vi "ADIS16448_CRC.vi"() -> (2 "CRC16-ADIS":u16, 10 "16-bit Array":i16[](array[numeric])=[15, -8, 10, -447, -52, 1110, 551, -605, -3054, -16068, -148])   [LabVIEW 2017]
panel:
  out "8-bit Array":u8[](array[numeric])
  # "This vi calculates a CRC16 check on data generated from an \nADIS16448 IMU when using burst mode (MSC_CTRL[4] = 1). \nThis implementation is a variant of the CCITT X.25 spec.\n\nJuan Chong - December 2017"
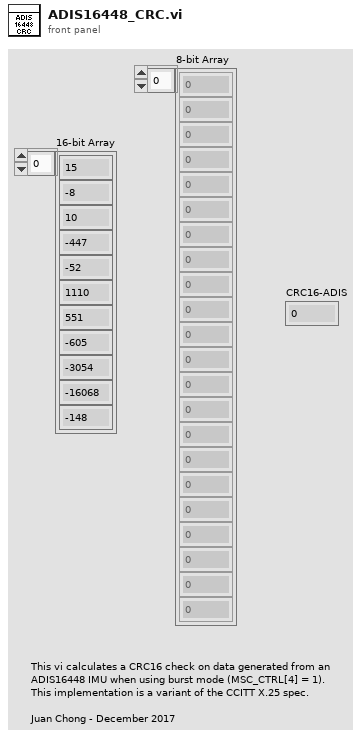
[diagram p1: front panel]
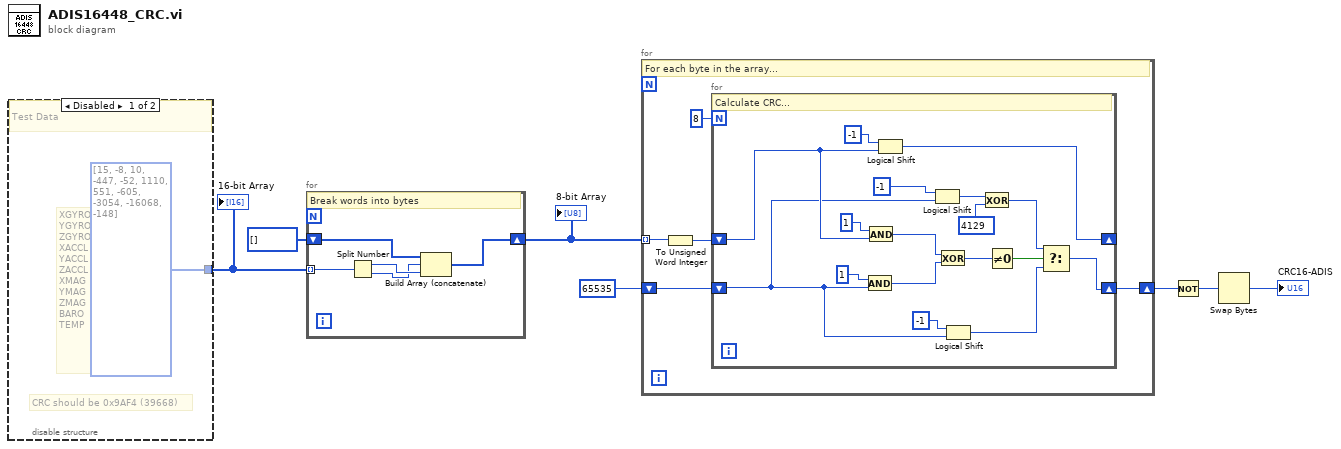
[diagram p0: block diagram]
diagram:
  n1 = disable-structure shown="Disabled" {
    disable-tunnel: [i16[] [15, -8, 10, -447, -52, 1110, 551, -605, -3054, -16068, -148] ("initialized array") _] -> w7
    frame Disabled {
      # "CRC should be 0x9AF4 (39668)"
      # "XGYRO\nYGYRO\nZGYRO\nXACCL\nYACCL\nZACCL\nXMAG\nYMAG\nZMAG\nBARO\nTEMP"
      # "Test Data"
    }
    frame Enabled {
    }
  }
  "16-bit Array" <- w7
  n2 = for {
    tunnel: w7 -> [w13] mode=indexing
    shift-right: [w12] -> w5
    shift-left: u8[] [] -> [w11]
    # "Break words into bytes"
    n3 = Split Number(x=w13) -> (hi(x)=w10:u8, lo(x)=w9:u8)
    n4 = Build Array (concatenate)(w11, w9, w10) -> (w12:u8[])
  }
  "8-bit Array" <- w5
  n5 = for {
    tunnel: w5 -> [w15] mode=indexing
    shift-right: [w17] -> w3
    shift-left: u16 65535 -> [w18]
    # "For each byte in the array..."
    n6 = To Unsigned Word Integer(number=w15) -> (unsigned 16bit integer=w14:u16)
    n7 = for {
      N: 8 -> [_]
      shift-right: [w25] -> w17
      shift-left: w18 -> [w19]
      shift-right: [w21] -> _
      shift-left: w14 -> [w20]
      # "Calculate CRC..."
      n8 = And(x=u16 1, y=w19) -> (x .and. y?=w34:u16)
      n9 = And(x=u16 1, y=w20) -> (x .and. y?=w23:u16)
      n10 = Logical Shift(y=i16 -1, x=w20) -> (x << y=w21:u16)
      n11 = Logical Shift(y=i16 -1, x=w19) -> (x << y=w30:u16)
      n12 = Exclusive Or(1:w34, 2:w23) -> (0:w33:u16)
      n13 = Logical Shift(y=i16 -1, x=w19) -> (x << y=w26:u16)
      n14 = Exclusive Or(1:u16 4129, 2:w30) -> (0:w28:u16)
      n15 = Not Equal To 0?(x=w33) -> (x != 0?=w32:bool)
      n16 = Select(t=w28, s=w32, f=w26) -> (s? t:f=w25:u16)
    }
  }
  n17 = Not(x=w3) -> (.not. x?=w2:u16)
  n18 = Swap Bytes(anything=w2) -> (byte swapped=→"CRC16-ADIS":u16)
